vi "Vypocet_spektra.vi"(0 "waveform":waveform(dbl)) -> (1 "Frekvence":i32, 2 "XY Graph":cluster{dbl[], dbl[]}(graph))   [LabVIEW 2019]
uses:
  <vilib>/Analysis/2dsp.llb/Real FFT.vi
  <vilib>/Analysis/NI_AALPro.lvlib
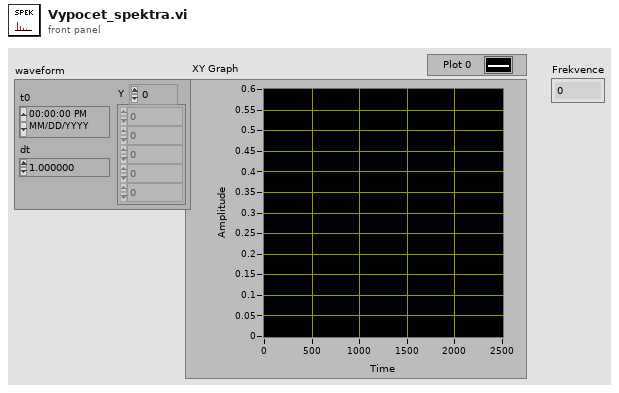
[diagram p1: front panel]
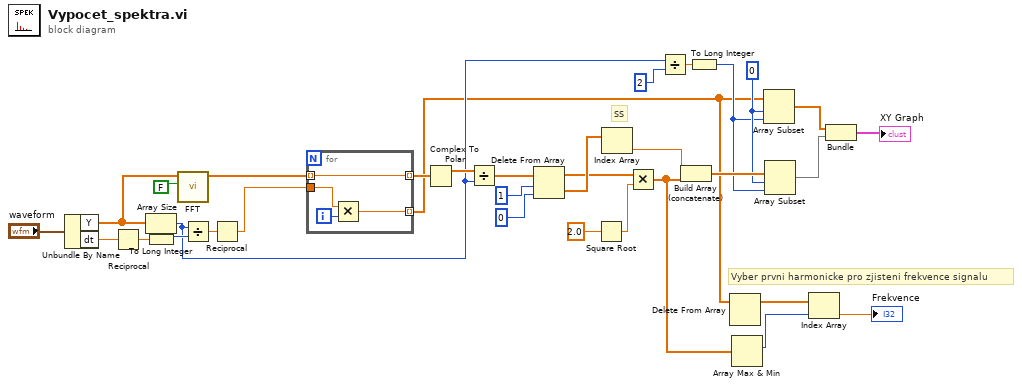
[diagram p0: block diagram]
diagram:
  w14 = 0
  # "Vyber prvni harmonicke pro zjisteni frekvence signalu"
  # "SS"
  n1 = Unbundle By Name("waveform") -> ("Y"=w28:dbl[], "dt"=w32:dbl)
  n2 = Reciprocal(x=w32) -> (1/x=w31:dbl)
  n3 = Array Size(array=w28) -> (size(s)=w6:i32)
  n4 = To Long Integer(number=w31) -> (32bit integer=w30:i32)
  n5 = call-poly <vilib>:"FFT.vi"("shift?"=FALSE, "X"=w28) -> ("FFT {X}"=w27:cdb[])  [unwired: 8 in, 1 out]
  n6 = Divide(x=w6, y=w30) -> (x/y=w29:dbl)
  n7 = Reciprocal(x=w29) -> (1/x=w26:dbl)
  n8 = for {
    tunnel: w27 -> [w34] mode=indexing
    tunnel: w26 -> [w36]
    tunnel: [w35] -> w4 mode=indexing
    tunnel: [w34] -> w25 mode=indexing
    i -> [w37]
    n9 = Multiply(x=w36, y=w37) -> (x*y=w35:dbl)
  }
  n10 = Complex To Polar(r * e^(i*theta)=w25) -> (r=w24:dbl[])  [unwired: 1 out]
  n11 = Divide(x=w24, y=w6) -> (x/y=w21:dbl[])
  n12 = Delete From Array(array=w21, length=1, index=0) -> (deleted portion=w20:dbl[], array with subset deleted=w19:dbl[])
  n13 = Square Root(x=2.0) -> (sqrt(x)=w18:dbl)
  n14 = Index Array(array=w20) -> (element=w16:dbl)  [unwired: 1 in]
  n15 = Multiply(x=w19, y=w18) -> (x*y=w5:dbl[])
  n16 = Divide(x=w6, y=2) -> (x/y=w12:dbl)
  n17 = Build Array (concatenate)(w16, w5) -> (w15:dbl[])
  n18 = To Long Integer(number=w12) -> (32bit integer=w11:i32)
  n19 = Delete From Array(array=w4) -> (array with subset deleted=w3:dbl[])  [unwired: 2 in, 1 out]
  n20 = Array Max & Min(array=w5) -> (max index (indices)=w2:i32)  [unwired: 3 out]
  n21 = Array Subset(array=w4, index=w14, length=w11) -> (w10:dbl[])
  n22 = Array Subset(array=w15, index=w14, length=w11) -> (w7:dbl[])
  n23 = Index Array(array=w3, index=w2) -> (element=→"Frekvence":dbl)
  n24 = Bundle(w10, w7) -> (→"XY Graph":cluster{dbl[], dbl[]})  [unwired: 1 in]
